vi "Random Color.vi"() -> (2 "Color":u32(colorbox))   [LabVIEW 2021, in "Dev Panel.lvclass"]
uses:
  Dev Panel.lvclass
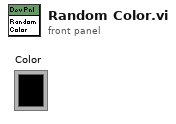
[diagram p1: front panel]
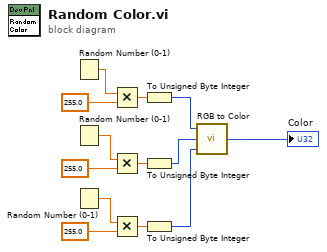
[diagram p0: block diagram]
diagram:
  n1 = Random Number (0-1)() -> (number: 0 to 1=w1:dbl)
  n2 = Random Number (0-1)() -> (number: 0 to 1=w9:dbl)
  n3 = Random Number (0-1)() -> (number: 0 to 1=w8:dbl)
  n4 = Multiply(x=w1, y=255.0) -> (x*y=w4:dbl)
  n5 = Multiply(x=w9, y=255.0) -> (x*y=w11:dbl)
  n6 = Multiply(x=w8, y=255.0) -> (x*y=w6:dbl)
  n7 = To Unsigned Byte Integer(number=w4) -> (unsigned 8bit integer=w5:u8)
  n8 = To Unsigned Byte Integer(number=w11) -> (unsigned 8bit integer=w12:u8)
  n9 = To Unsigned Byte Integer(number=w6) -> (unsigned 8bit integer=w13:u8)
  n10 = call <vilib>:"RGB to Color.vi"("B"=w13, "G"=w12, "R"=w5) -> ("Color"=→"Color":u32)
